vi "LoopTimer.vi"() -> (3 "Loop time (s)":dbl)   [LabVIEW 2020]
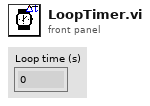
[diagram p1: front panel]
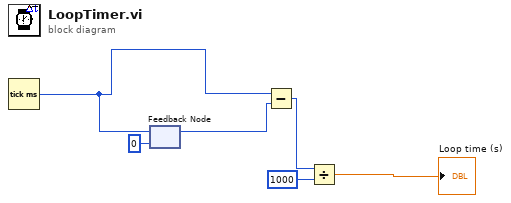
[diagram p0: block diagram]
diagram:
  n1 = Tick Count (ms)() -> (millisecond timer value=w2:u32)
  n2 = feedback #1(u32 0 ("millisecond timer value")) -> (w3:u32)
  n3 = feedback-in #1(w2) -> ()
  n4 = Subtract(x=w2, y=w3) -> (x-y=w4:u32)
  n5 = Divide(x=w4, y=u32 1000) -> (x/y=→"Loop time (s)":dbl)
